vi "Query Output Protection Status.vi"(8 "error in":errorcluster, 11 "VISA resource name":refnum<visa-resource-name>) -> (0 "error out":errorcluster, 1 "OCP Tripped State":bool, 2 "OVP Tripped State":bool, 3 "VISA resource name out":refnum<visa-resource-name>)   [LabVIEW 2015, in "IT6700H.lvlib"]
doc: "Returns over voltage protection (OVP) and over current protection (OCP) status for a desired channel."
uses:
  <instrlib>/IT6700H/IT6700H.lvlib
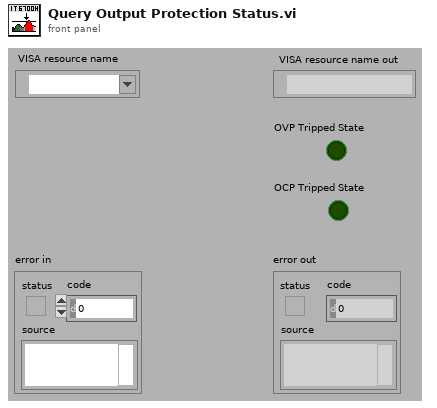
[diagram p1: front panel]
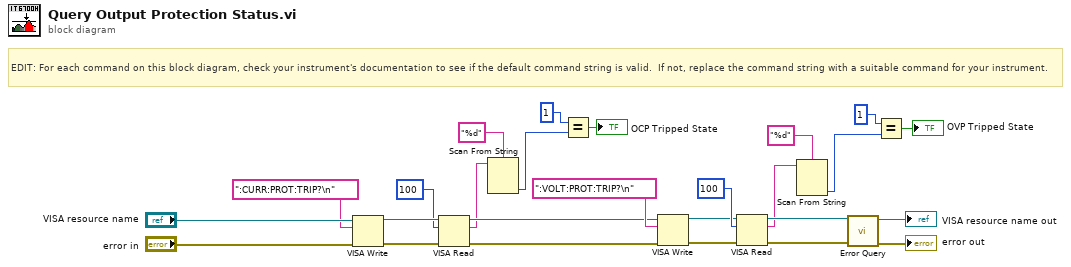
[diagram p0: block diagram]
diagram:
  # "EDIT: For each command on this block diagram, check your instrument's documentation to see if the default command string is valid.  If not, replace the command string with a suitable command for your instrument."
  n1 = VISA Write(VISA resource name="VISA resource name", write buffer=":CURR:PROT:TRIP?\n", error in (no error)="error in") -> (VISA resource name out=w20:refnum<visa-resource-name>, error out=w21:errorcluster)  [unwired: 1 out]
  n2 = VISA Read(VISA resource name=w20, byte count=u32 100, error in (no error)=w21) -> (VISA resource name out=w12:refnum<visa-resource-name>, read buffer=w8:string, error out=w11:errorcluster)  [unwired: 1 out]
  n3 = Scan From String(format string="%d", input string=w8) -> (output 1=w2:i32)  [unwired: 3 in, 3 out]
  n4 = Equal?(x=1, y=w2) -> (x = y?=→"OCP Tripped State":bool)
  n5 = VISA Write(VISA resource name=w12, write buffer=":VOLT:PROT:TRIP?\n", error in (no error)=w11) -> (VISA resource name out=w16:refnum<visa-resource-name>, error out=w15:errorcluster)  [unwired: 1 out]
  n6 = VISA Read(VISA resource name=w16, byte count=u32 100, error in (no error)=w15) -> (VISA resource name out=w10:refnum<visa-resource-name>, read buffer=w4:string, error out=w9:errorcluster)  [unwired: 1 out]
  n7 = Scan From String(format string="%d", input string=w4) -> (output 1=w1:i32)  [unwired: 3 in, 3 out]
  n8 = call <instrlib>:"Error Query.vi"("error in"=w9, "VISA resource name"=w10) -> ("error out"=→"error out":errorcluster, "VISA resource name out"=→"VISA resource name out":refnum<visa-resource-name>)  [unwired: 6 in, 2 out]
  n9 = Equal?(x=1, y=w1) -> (x = y?=→"OVP Tripped State":bool)
